vi "eFGV - Sampling Rate.vi"(6 "eFGV States":T1, 8 "Error In":errorcluster, 11 "Sampling Rate":i32) -> (0 "Error Out":errorcluster, 2 "Event Sampling Rate":refnum<user-event>, 3 "Sampling Rate Out":i32)   [LabVIEW 2020]
uses:
  Control/State - eFGV.ctl
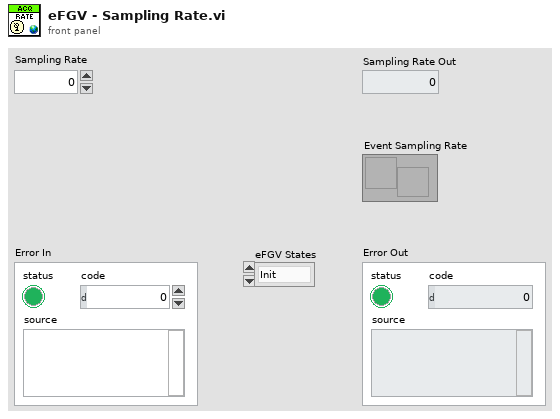
[diagram p1: front panel]
types:
  T1 = typedef "State - eFGV.ctl" = enum16{"Init", "Read", "Write", "Exit"}
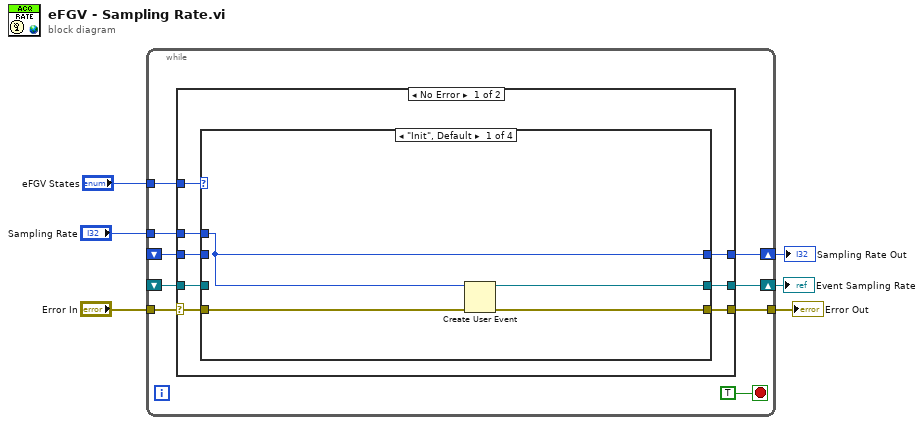
[diagram p0: block diagram]
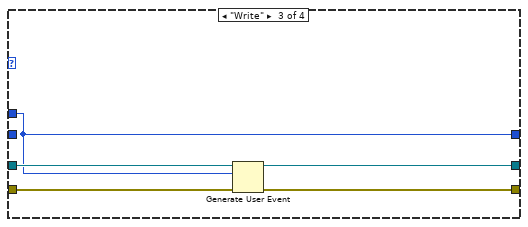
[diagram p3: hidden frame]
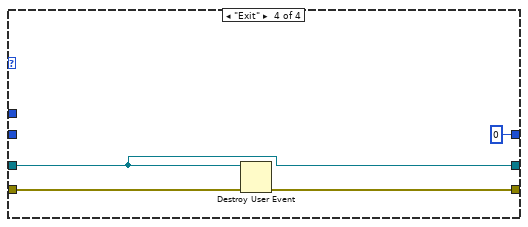
[diagram p4: hidden frame]
diagram:
  n1 = while {
    tunnel: "eFGV States" -> [w12]
    tunnel: "Error In" -> [w15]
    tunnel: [w14] -> w5
    tunnel: "Sampling Rate" -> [w11]
    shift-right: [w10] -> w1
    shift-left: _ -> [w9]
    shift-right: [w8] -> w2
    shift-left: _ -> [w7]
    stop <- TRUE stop-if-true
    n2 = case shown="No Error" w15 {
      selector: w15 -> [w23 w42]
      tunnel: w12 -> [w21 _]
      tunnel: [w22 w42] -> w14
      tunnel: w11 -> [w20 _]
      tunnel: [w19 w41] -> w10
      tunnel: w9 -> [w18 w41]
      tunnel: [w17 w40] -> w8
      tunnel: w7 -> [w16 w40]
      frame No Error {
        n3 = case shown="\"Init\", Default" w21 {
          tunnel: w23 -> [w27 w30 w35 w39]
          tunnel: [w26 w30 w34 w38] -> w22
          tunnel: w20 -> [w24 _ w31 _]
          tunnel: [w25 w29 w32 w37] -> w19
          tunnel: w18 -> [_ w29 w33 w37]
          tunnel: [w24 w28 w31 0 ("Acquisition Rate")] -> w17
          tunnel: w16 -> [_ w28 _ _]
          frame "Init", Default {
            n4 = Create User Event(user event datatype=w24, error in=w27) -> (user event=w25:refnum<user-event>, error out=w26:errorcluster)
          }
          frame "Read" {
          }
          frame "Write" {
            n5 = Generate User Event(user event=w33, event data cluster=w31, error in=w35) -> (user event out=w32:refnum<user-event>, error out=w34:errorcluster)  [unwired: 1 in]
          }
          frame "Exit" {
            n6 = Destroy User Event(user event=w37, error in=w39) -> (error out=w38:errorcluster)
          }
        }
      }
      frame Error {
      }
    }
  }
  "Error Out" <- w5
  "Sampling Rate Out" <- w2
  "Event Sampling Rate" <- w1
